vi "CMN_TimeStamp2Seconds.vi"(8 "DST":bool, 9 "TimeStamp string (yyyy-mm-ddThh:mm:ss)":string) -> (1 "date time rec out":T1, 2 "seconds out":dbl format="%.1f")   [LabVIEW 2016]
panel:
  in  "date time rec":T1
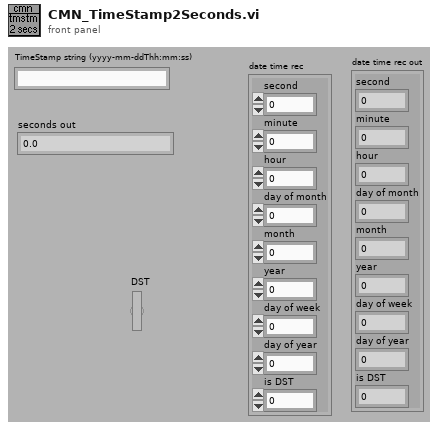
[diagram p1: front panel]
types:
  T1 = cluster{"second":i32, "minute":i32, "hour":i32, "day of month":i32, "month":i32, "year":i32, "day of week":i32, "day of year":i32, "is DST":i32}
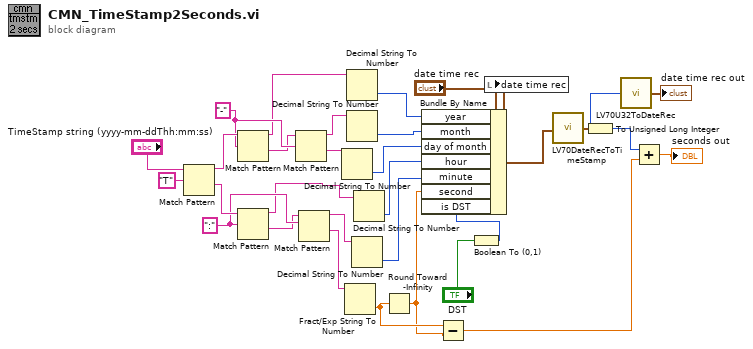
[diagram p0: block diagram]
diagram:
  w15 = ":" ("regular expression")
  w26 = "-" ("regular expression")
  n1 = Match Pattern(string="TimeStamp string (yyyy-mm-ddThh:mm:ss)", regular expression="T") -> (before substring=w27:string, after substring=w16:string)  [unwired: 3 out]
  n2 = Match Pattern(string=w27, regular expression=w26) -> (before substring=w22:string, after substring=w23:string)  [unwired: 3 out]
  n3 = Match Pattern(string=w16, regular expression=w15) -> (before substring=w13:string, after substring=w14:string)  [unwired: 3 out]
  n4 = Match Pattern(string=w23, regular expression=w26) -> (before substring=w24:string, after substring=w25:string)  [unwired: 3 out]
  n5 = Match Pattern(string=w14, regular expression=w15) -> (before substring=w12:string, after substring=w11:string)  [unwired: 1 in, 2 out]
  n6 = Decimal String To Number(string=w25) -> (number=w19:i32)  [unwired: 3 out]
  n7 = Fract/Exp String To Number(string=w11) -> (number=w5:dbl)  [unwired: 4 out]
  n8 = Decimal String To Number(string=w22) -> (number=w21:i32)  [unwired: 3 out]
  n9 = Decimal String To Number(string=w24) -> (number=w20:i32)  [unwired: 3 out]
  n10 = Decimal String To Number(string=w12) -> (number=w9:i32)  [unwired: 3 out]
  n11 = Decimal String To Number(string=w13) -> (number=w10:i32)  [unwired: 3 out]
  n12 = Round Toward -Infinity(1:w5) -> (0:w4:dbl)
  n13 = Subtract(x=w5, y=w4) -> (x-y=w6:dbl)
  n14 = Boolean To (0,1)(Boolean="DST") -> (0, 1=w2:i16)
  n15 = Bundle By Name(cluster="date time rec", "year"=w21, "month"=w20, "day of month"=w19, "hour"=w10, "minute"=w9, "second"=w4, "is DST"=w2) -> (w18:T1)
  n16 = local write "date time rec"(w18) -> ()
  n17 = call <vilib>:"LV70DateRecToTimeStamp.vi"("date time rec"=w18) -> ("Time Stamp"=w1:timestamp)
  n18 = To Unsigned Long Integer(number=w1) -> (unsigned 32bit integer=w7:u32)
  n19 = call <vilib>:"LV70U32ToDateRec.vi"("Time"=w7) -> ("date time rec"=→"date time rec out":T1)
  n20 = Add(x=w7, y=w6) -> (x+y=→"seconds out":dbl)
